vi "Control-Relay-board-with-Arduino.vi"(0 "Select Com Port":refnum<visa-resource-name>, 5 "Relay Open Close":bool, 11 "error In":errorcluster) -> (4 "return count":u32, 6 "Output String":string, 15 "error Out":errorcluster)   [LabVIEW 2020]
uses:
  <vilib>/Instr/_visa.llb/VISA Set IO Buffer Mask.ctl
  <vilib>/Instr/_visa.llb/VISA Flush IO Buffer Mask.ctl
  <vilib>/Instr/_visa.llb/VISA Configure Serial Port (Instr).vi
panel:
  out "Number of Bytes at Serial Port":u32
  # "True is Close\nFalse is Open (Default)"
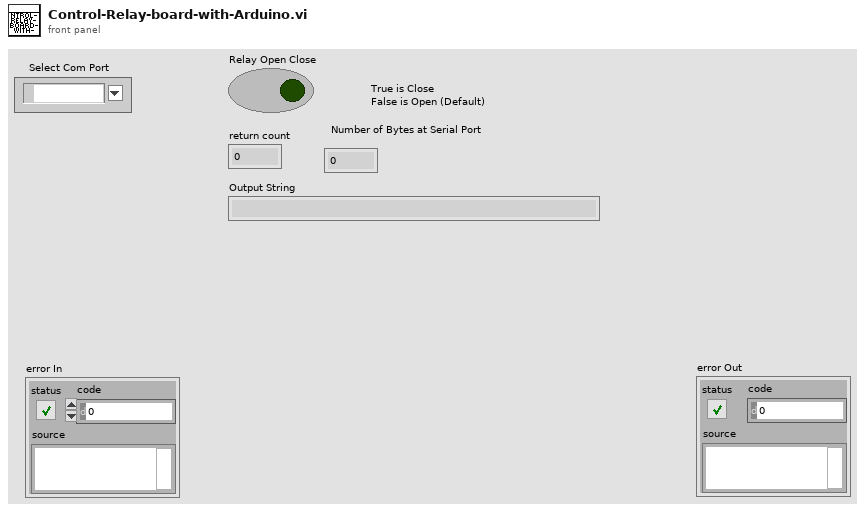
[diagram p1: front panel]
types:
  T1 = enum16{"Native", "Native Command Line", "UNIX", "Macintosh", "DOS"}
  T2 = typedef "VISA Flush IO Buffer Mask.ctl" = u16
  T3 = typedef "VISA Set IO Buffer Mask.ctl" = u16
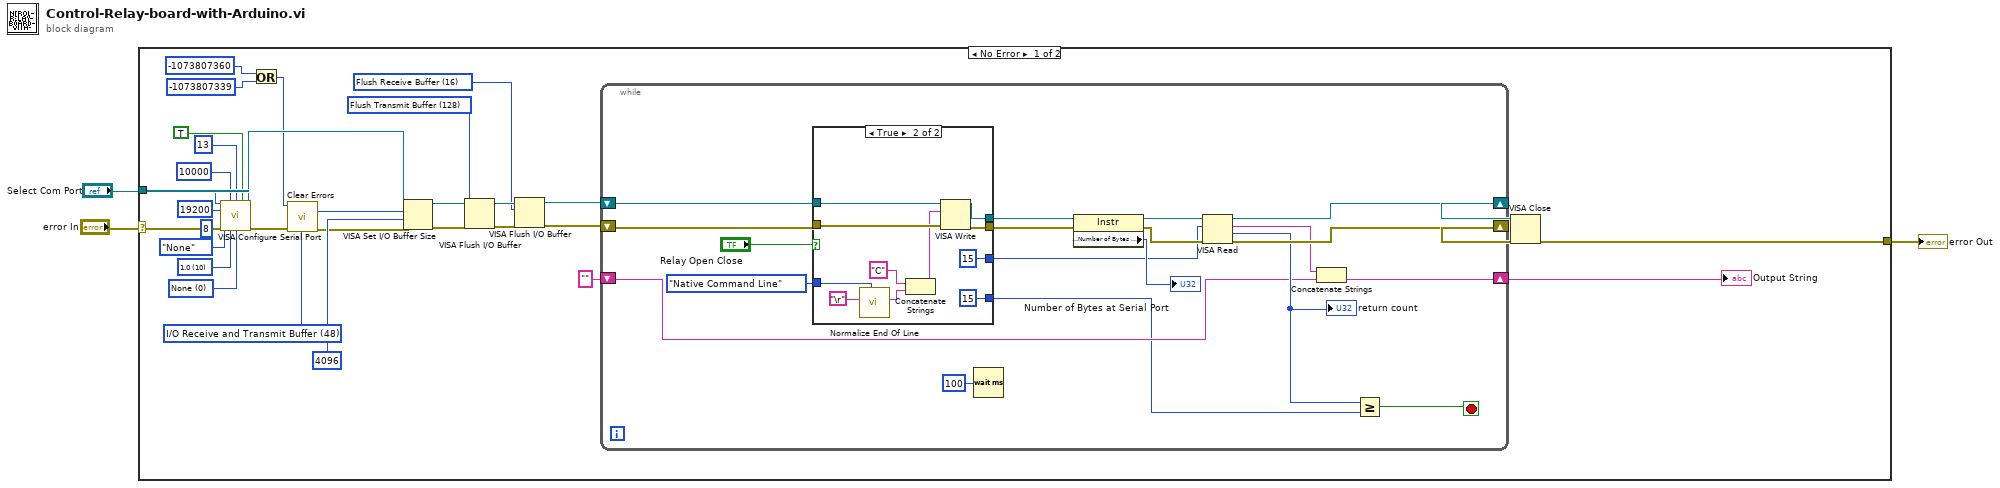
[diagram p0: block diagram]
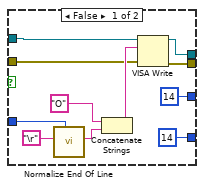
[diagram p2: hidden frame]
diagram:
  n1 = case shown="No Error" "error In" {
    selector: "error In" -> [w34 w76]
    tunnel: [w22 w76] -> w2
    tunnel: "Select Com Port" -> [w33 _]
    frame No Error {
      w7 = T2 16 items=["Flush Receive Buffer"=16, "Write Transmit Buffer to Device"=32, "Flush Receive Buffer (No I/O)"=64, "Flush Transmit Buffer"=128] ("Mask")
      w10 = T2 128 items=["Flush Receive Buffer"=16, "Write Transmit Buffer to Device"=32, "Flush Receive Buffer (No I/O)"=64, "Flush Transmit Buffer"=128] ("Mask")
      w26 = T3 48 items=["I/O Receive Buffer"=16, "I/O Transmit Buffer"=32, "I/O Receive and Transmit Buffer"=48] ("Mask")
      w28 = u16 0 items=["None", "XON/XOFF", "RTS/CTS", "XON/XOFF & RTS/CTS", "DTR/DSR", "XON/XOFF & DTR/DSR"] ("flow control (0:none)")
      w29 = u16 10 items=["1.0"=10, "1.5"=15, "2.0"=20] ("stop bits (10: 1 bit)")
      n2 = call-poly "VISA Configure Serial Port"("VISA resource name"=w33, "timeout (10sec)"=u32 10000, "termination char\n(0xA = '\\n' = LF)"=u8 13 ("termination char\n(0xA = '\\n' = LF)"), "Enable Termination\nChar (T)"=TRUE ("Enable Termination\nChar (T)"), "baud rate (9600)"=u32 19200, "data bits (8)"=u16 8, "parity (0:none)"=enum16{"None", "Odd", "Even", "Mark", "Space"}."None", "error in (no error)"=w34, "stop bits (10: 1 bit)"=w29, "flow control (0:none)"=w28) -> ("VISA resource name out"=w27:refnum<visa-resource-name>, "error out"=w19:errorcluster)  [unwired: 4 in]
      n3 = Or(x=-1073807360 ("specific error code to clear (0: all)"), y=-1073807339 ("specific error code to clear (0: all)")) -> (x .or. y?=w14:i32)
      n4 = call <vilib>:"Clear Errors.vi"("error in (no error)"=w19, "specific error code to clear (0: all)"=w14) -> ("error out"=w13:errorcluster)  [unwired: 4 in, 1 out]
      n5 = VISA Set I/O Buffer Size(VISA resource name=w27, mask (16)=w26, size (4096)=u32 4096, error in (no error)=w13) -> (VISA resource name out=w12:refnum<visa-resource-name>, error out=w11:errorcluster)
      n6 = VISA Flush I/O Buffer(VISA resource name=w12, mask (16)=w10, error in (no error)=w11) -> (VISA resource name out=w8:refnum<visa-resource-name>, error out=w9:errorcluster)
      n7 = VISA Flush I/O Buffer(VISA resource name=w8, mask (16)=w7, error in (no error)=w9) -> (VISA resource name out=w5:refnum<visa-resource-name>, error out=w6:errorcluster)
      n8 = while {
        shift-right: [w49] -> w23
        shift-left: w6 -> [w35]
        shift-right: [w50] -> w24
        shift-left: w5 -> [w36]
        shift-right: [w40] -> w17
        shift-left: "" -> [w41]
        stop <- w42 stop-if-true
        n9 = case shown="True" "Relay Open Close" {
          tunnel: w36 -> [w57 w75]
          tunnel: w35 -> [w60 w74]
          tunnel: T1."Native Command Line" ("end of line (Native)") -> [w56 w71]
          tunnel: [w59 w68] -> w52
          tunnel: [w58 w67] -> w51
          tunnel: [u32 14 ("byte count") u32 15 ("byte count")] -> w38
          tunnel: [u32 14 ("y") u32 15 ("y")] -> w37
          frame False {
            n10 = call <vilib>:"Normalize End Of Line.vi"("end of line (Native)"=w56, "string in"="\r") -> ("string out"=w63:string)  [unwired: 6 in]
            n11 = Concatenate Strings("O" ("string"), w63) -> (w64:string)
            n12 = VISA Write(VISA resource name=w57, write buffer=w64, error in (no error)=w60) -> (VISA resource name out=w58:refnum<visa-resource-name>, error out=w59:errorcluster)  [unwired: 1 out]
          }
          frame True {
            n13 = call <vilib>:"Normalize End Of Line.vi"("end of line (Native)"=w71, "string in"="\r") -> ("string out"=w73:string)  [unwired: 6 in]
            n14 = Concatenate Strings("C" ("string"), w73) -> (w69:string)
            n15 = VISA Write(VISA resource name=w75, write buffer=w69, error in (no error)=w74) -> (VISA resource name out=w67:refnum<visa-resource-name>, error out=w68:errorcluster)  [unwired: 1 out]
          }
        }
        n16 = Wait (ms)(milliseconds to wait=u32 100) -> ()  [unwired: 1 out]
        n17 = property class="Instr"(reference=w51, error in=w52) -> (reference out=w47:refnum<visa-resource-name>, error out=w46:errorcluster, "Serial Settings:Number of Bytes at Serial Port"=→"Number of Bytes at Serial Port":u32)
        n18 = VISA Read(VISA resource name=w47, byte count=w38, error in (no error)=w46) -> (VISA resource name out=w50:refnum<visa-resource-name>, read buffer=w45:string, return count=w44:u32, error out=w49:errorcluster)
        "return count" <- w44
        n19 = Concatenate Strings(w45, w41) -> (w40:string)
        n20 = Greater Or Equal?(x=w44, y=w37) -> (x >= y?=w42:bool)
      }
      "Output String" <- w17
      n21 = VISA Close(VISA resource name=w24, error in (no error)=w23) -> (error out=w22:errorcluster)
    }
    frame Error {
    }
  }
  "error Out" <- w2
